vi "追溯全部变量.vi"() -> ()   [LabVIEW 2020]
panel:
  in  "工件状态":string
  in  "不合格代码":string[](array[string])
  in  "质量信息":string[][](table)
  in  "物料信息":string[][](table)
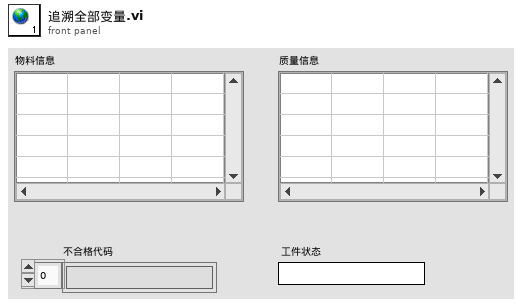
[diagram p1: front panel]
diagram:
